vi "Iterator.vi"(1 "Reset":bool) -> (0 "i":i32)   [LabVIEW 2020, in "ArduinoSerialBling.lvlib"]
uses:
  ArduinoSerialBling.lvlib
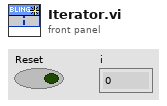
[diagram p1: front panel]
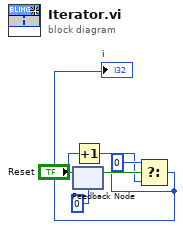
[diagram p0: block diagram]
diagram:
  n1 = feedback #1(0) -> (w2:i32)
  n2 = Increment(x=w2) -> (x+1=w3:i32)
  n3 = Select(t=0, s="Reset", f=w3) -> (s? t:f=w5:i32)
  "i" <- w5
  n4 = feedback-in #1(w5) -> ()
